vi "espacion_de_estado_continuo.vi"(0 "A":T1=[[-2.0, -1.0], [1.0, 0.0]], 1 "B":dbl[](array[numeric])=[1.0, 0.0], 2 "C":dbl[](array[numeric])=[1.0, 2.0], 3 "dX(t)":dbl[](array[numeric]) format="%.2f", 4 "u(t)":dbl) -> (5 "y(t)":dbl, 6 "X(t)":dbl[](array[numeric]) format="%.2f")   [LabVIEW 2018]
uses:
  <vilib>/Analysis/Matrix/Datatypes/RealMatrix.ctl
  <vilib>/Analysis/baseanly.llb/Real Dot Product.vi
  <vilib>/Analysis/baseanly.llb/A x Vector.vi
  IAControl Library/continuous linear.llb/Integrator (DBL Array).vi
  <vilib>/Analysis/NI_AALBase.lvlib
  <vilib>/Analysis/Matrix/NI_Matrix.lvlib
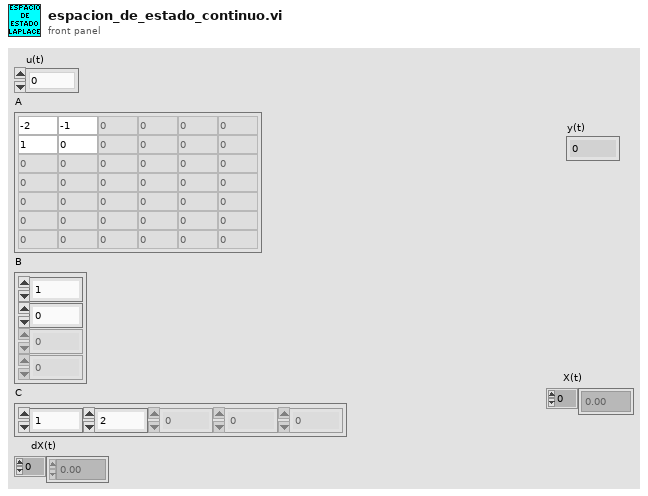
[diagram p1: front panel]
types:
  T1 = typedef "NI_Matrix.lvlib/RealMatrix.ctl" = dbl[][]
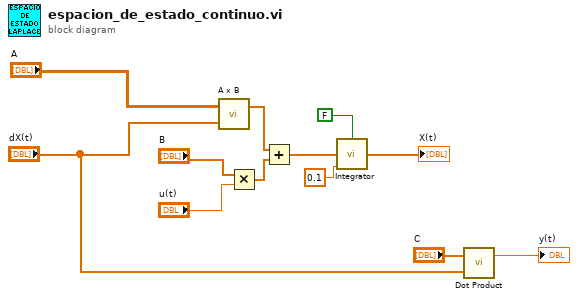
[diagram p0: block diagram]
diagram:
  n1 = call-poly <vilib>:"A x B.vi"("Vector"="dX(t)", "A"="A") -> ("A x Vector"=w11:dbl[])  [unwired: 1 out]
  n2 = Multiply(x="B", y="u(t)") -> (x*y=w12:dbl[])
  n3 = Add ("Add.vi")(x=w11, y=w12) -> (x+y=w10:dbl[])
  n4 = call-poly "Integrator.vi"("initialize"=FALSE, "input points"=w10, "dt"=0.1) -> ("output points"=→"X(t)":dbl[])  [unwired: 12 in]
  n5 = call-poly <vilib>:"Dot Product.vi"("Y Vector"="dX(t)", "X Vector"="C") -> ("X * Y"=→"y(t)":dbl)  [unwired: 1 out]
